vi "Main.vi"() -> ()   [LabVIEW 2019]
uses:
  View/MainPage/MainPage/MainPage.lvclass
  D:/Program Files (x86)/National Instruments/LabVIEW 2019/vi.lib/ActorFramework/Actor/Actor.lvclass
  <vilib>/ActorFramework/Actor/Actor.lvclass
panel:
  in  "MainPage.lvlib:MainPage.lvclass":refnum<class "MainPage.lvclass">
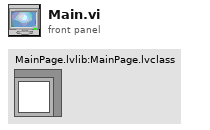
[diagram p1: front panel]
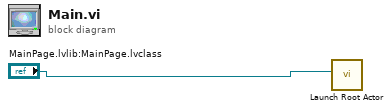
[diagram p0: block diagram]
diagram:
  n1 = call <vilib>:"Launch Root Actor.vi"("Actor"="MainPage.lvlib:MainPage.lvclass") -> ()  [unwired: 9 in, 2 out]
